vi "SIMULATE.vi"(8 "error in (no error)":errorcluster, 11 "FPGA_Sim":refnum<class "FPGA_Mock.lvclass">) -> (0 "error out":errorcluster, 3 "FPGA_Sim 2":refnum<class "FPGA_Mock.lvclass">)   [LabVIEW 2019, in "FPGA_Mock.lvclass"]
uses:
  FPGA_Mock.lvclass
  FPGA_Mock.lvclass/FPGA_Mock.ctl
panel:
  out "AO":dbl[](array[numeric])
  in  "Tab Control":enum32{"Channel testing", "HI Pressure testing"}(tab)=enum."HI Pressure testing"
  in  "DI":bool[](array[boolean])=[FALSE, FALSE, FALSE, FALSE, FALSE, FALSE, FALSE, FALSE, FALSE, FALSE, FALSE, FALSE, FALSE, FALSE, FALSE, FALSE, FALSE, FALSE, FALSE, FALSE, FALSE, FALSE, FALSE, FALSE, FALSE, FALSE, FALSE, FALSE, FALSE, FALSE, FALSE, FALSE]
  in  "AI":dbl[](array[numeric])=[1.0, 2.0, 3.0, 4.0, 5.0, 6.0, 7.0, 8.0, 9.0, 10.0, 11.0, 12.0, 13.0, 14.0, 15.0, 16.0]
  out "DO":bool[](array[boolean])
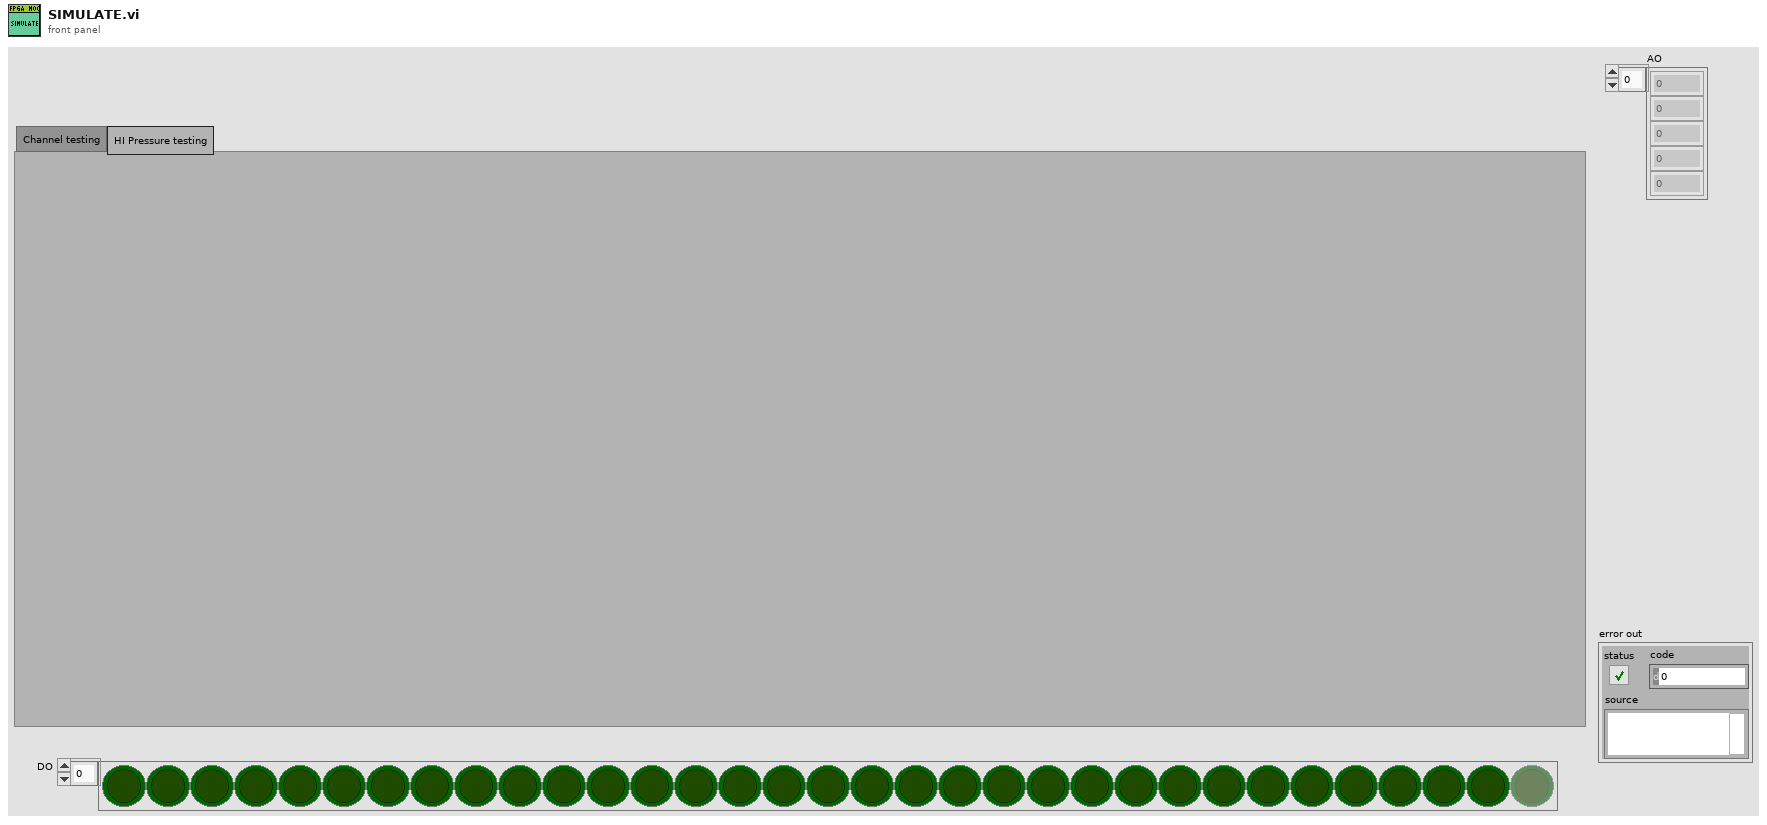
[diagram p1: front panel]
types:
  T1 = typedef "FPGA_Mock.lvclass/SharedData.ctl" = cluster{"DI":bool[], "DO":bool[], "AO":dbl[]}
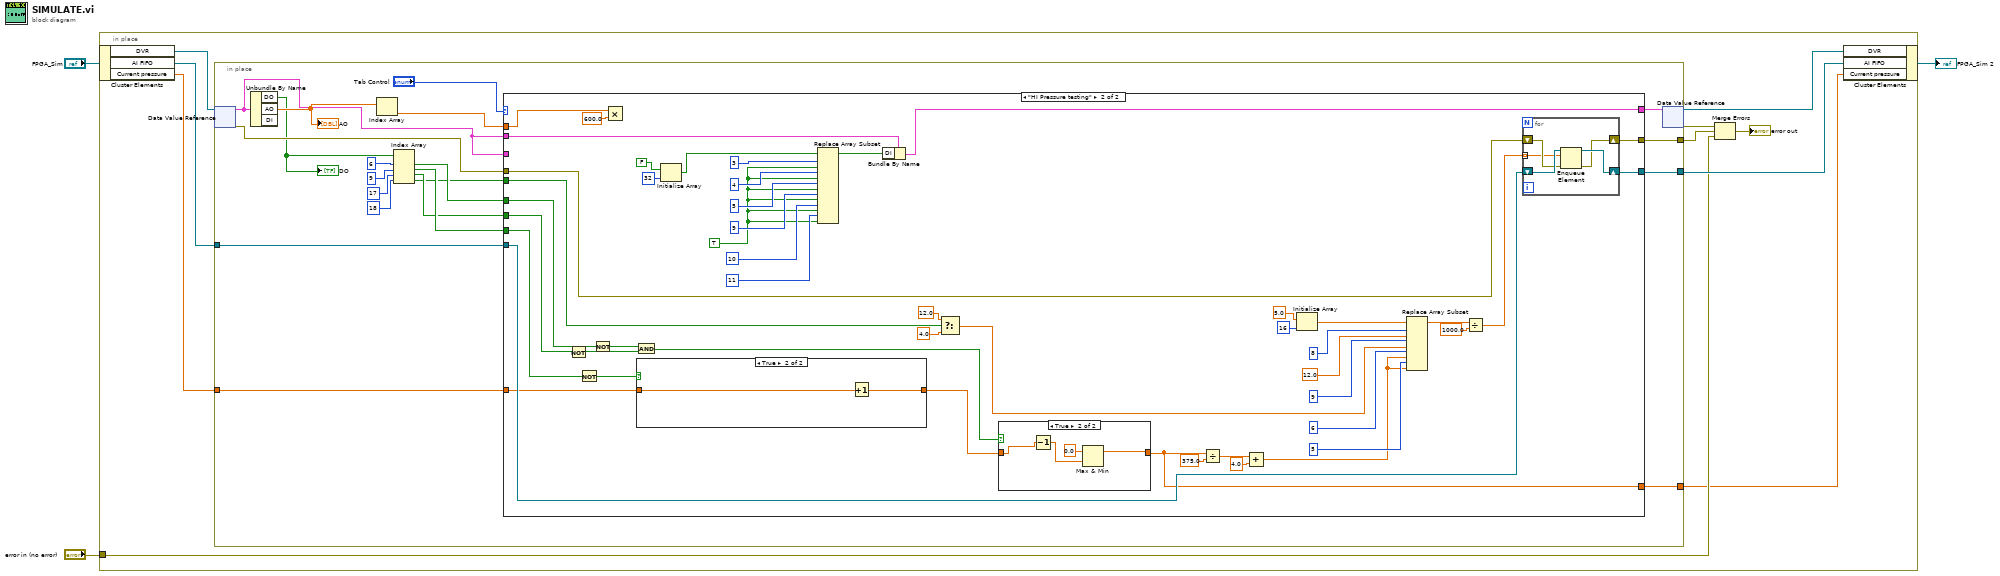
[diagram p0: block diagram]
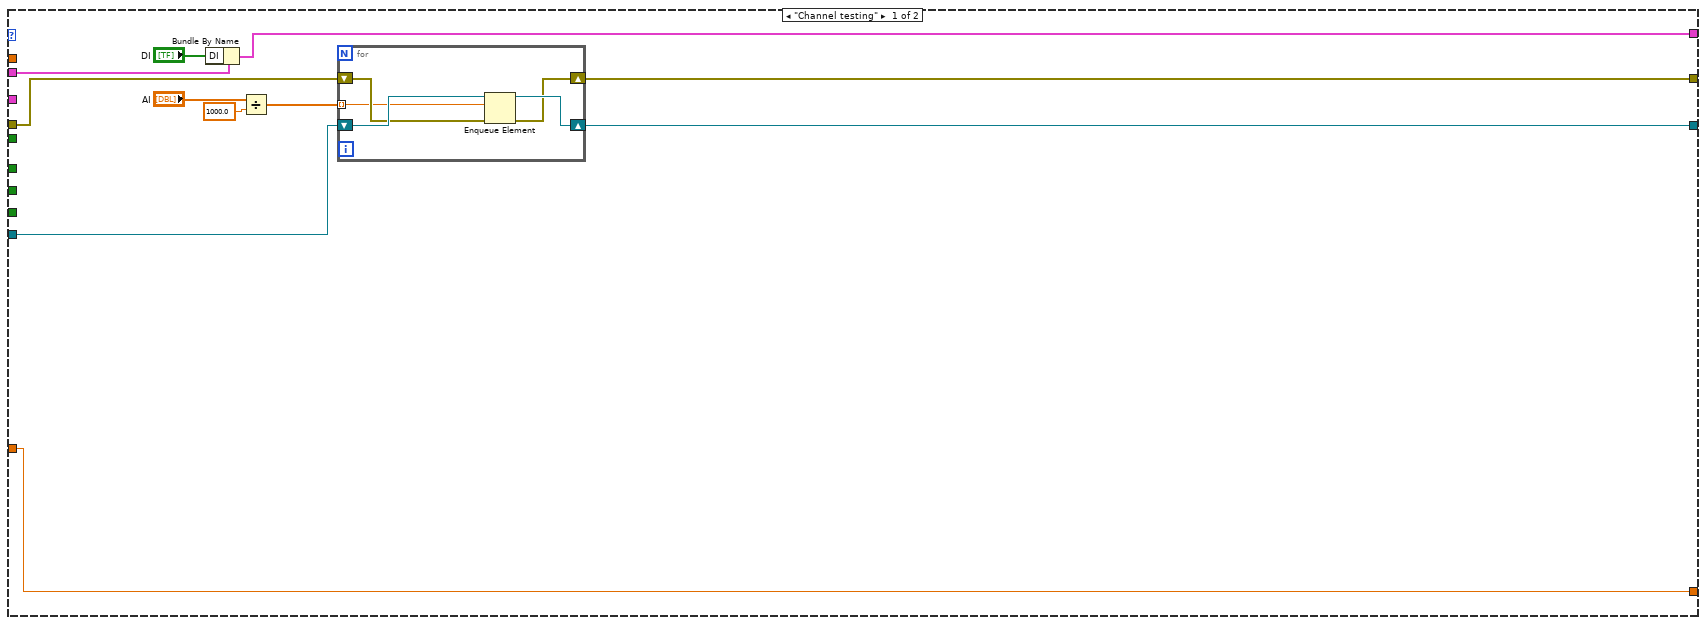
[diagram p2: hidden frame]
diagram:
  n1 = in-place {
    in-place-border: "error in (no error)" -> [w6]
    n2 = in-place-cluster #1("FPGA_Sim") -> ("DVR"=w13:refnum<data-value>, "AI FIFO"=w9:refnum<queue>, "Current pressure"=w5:dbl)
    n3 = in-place {
      in-place-border: w9 -> [w32]
      in-place-border: [w30] -> w8
      in-place-border: [w28] -> w7
      in-place-border: w5 -> [w15]
      in-place-border: [w14] -> w4
      n4 = in-place-dvr #2(w13) -> (w27:T1, w31:errorcluster)
      n5 = Unbundle By Name(w27) -> ("DO"=w24:bool[], "AO"=w26:dbl[])  [unwired: 1 out]
      "DO" <- w24
      "AO" <- w26
      n6 = Index Array(array=w26) -> (element=w25:dbl)  [unwired: 1 in]
      n7 = Index Array(array=w24, index #1=6 ("index"), index #2=9 ("index"), index #3=17 ("index"), index #4=18 ("index")) -> (element #1=w19:bool, element #2=w18:bool, element #3=w17:bool, element #4=w16:bool)
      n8 = case shown="\"HI Pressure testing\"" "Tab Control" {
        tunnel: w27 -> [w44 w97]
        tunnel: [w43 w77] -> w33
        tunnel: w32 -> [w38 w94]
        tunnel: w31 -> [w37 w93]
        tunnel: [w36 w92] -> w30
        tunnel: [w35 w91] -> w28
        tunnel: w27 -> [_ _]
        tunnel: w25 -> [_ w85]
        tunnel: w19 -> [_ w74]
        tunnel: w18 -> [_ w76]
        tunnel: w17 -> [_ w73]
        tunnel: w16 -> [_ w81]
        tunnel: w15 -> [w34 w75]
        tunnel: [w34 w68] -> w14
        frame "Channel testing" {
          n9 = Bundle By Name(cluster=w44, "DI"="DI") -> (w43:T1)
          n10 = Divide(x="AI", y=1000.0) -> (x/y=w40:dbl[])
          n11 = for {
            shift-right: [w48] -> w35
            shift-left: w38 -> [w49]
            shift-right: [w46] -> w36
            shift-left: w37 -> [w47]
            tunnel: w40 -> [w45] mode=indexing
            n12 = Enqueue Element(queue=w49, element=w45, error in (no error)=w47) -> (queue out=w48:refnum<queue>, error out=w46:errorcluster)  [unwired: 1 in, 1 out]
          }
        }
        frame "HI Pressure testing" {
          w56 = TRUE ("new element/subarray")
          n13 = Not(x=w73) -> (.not. x?=w50:bool)
          n14 = Not(x=w76) -> (.not. x?=w52:bool)
          n15 = Not(x=w74) -> (.not. x?=w51:bool)
          n16 = Multiply(x=w85, y=600.0) -> ()  [unwired: 1 out]
          n17 = And(x=w51, y=w50) -> (x .and. y?=w72:bool)
          n18 = case shown="True" w52 {
            tunnel: w75 -> [w103 w105]
            tunnel: [w103 w104] -> w71
            frame False {
            }
            frame True {
              n19 = Increment(x=w105) -> (x+1=w104:dbl)
            }
          }
          n20 = Initialize Array(FALSE ("new element/subarray"), 32 ("dimension size")) -> (w53:bool[])
          n21 = Replace Array Subset(array=w53, new element #1=w56, index #1=3 ("index"), new element #2=w56, index #2=4 ("index"), new element #3=w56, index #3=5 ("index"), new element #4=w56, index #4=9 ("index"), new element #5=w56, index #5=10 ("index"), new element #6=w56, index #6=11 ("index")) -> (w63:bool[])
          n22 = Bundle By Name(cluster=w97, "DI"=w63) -> (w77:T1)
          n23 = Select(t=12.0, s=w81, f=4.0) -> (s? t:f=w78:dbl)
          n24 = case shown="True" w72 {
            tunnel: w71 -> [w98 w102]
            tunnel: [w98 w99] -> w68
            frame False {
            }
            frame True {
              n25 = Decrement(x=w102) -> (x-1=w100:dbl)
              n26 = Max & Min(x=0.0, y=w100) -> (max(x,y)=w99:dbl)  [unwired: 1 out]
            }
          }
          n27 = Divide(x=w68, y=375.0) -> (x/y=w66:dbl)
          n28 = Add(x=w66, y=4.0) -> (x+y=w64:dbl)
          n29 = Initialize Array(5.0 ("element"), 16 ("dimension size")) -> (w88:dbl[])
          n30 = Replace Array Subset(array=w88, new element #1=12.0 ("new element/subarray"), index #1=8 ("index"), new element #2=w78, index #2=9 ("index"), new element #3=w64, index #3=6 ("index"), new element #4=w64, index #4=5 ("index")) -> (w87:dbl[])
          n31 = Divide(x=w87, y=1000.0) -> (x/y=w96:dbl[])
          n32 = for {
            shift-right: [w109] -> w91
            shift-left: w94 -> [w110]
            shift-right: [w107] -> w92
            shift-left: w93 -> [w108]
            tunnel: w96 -> [w106] mode=indexing
            n33 = Enqueue Element(queue=w110, element=w106, error in (no error)=w108) -> (queue out=w109:refnum<queue>, error out=w107:errorcluster)  [unwired: 1 in, 1 out]
          }
        }
      }
      n34 = in-place-dvr #2(w33) -> (w12:refnum<data-value>, w11:errorcluster)
    }
    n35 = Merge Errors(w11, w8, w6) -> (→"error out":errorcluster)
    n36 = in-place-cluster #1("DVR"=w12, "AI FIFO"=w7, "Current pressure"=w4) -> (→"FPGA_Sim 2":refnum<class "FPGA_Mock.lvclass">)
  }
